vi "Measure.vi"(8 "error in (no error)":errorcluster, 9 "Progress Ref":refnum<vi>, 10 "XY Graph Reference":refnum<vi>, 11 "AM-AM in":refnum<class "AM-AM.lvclass">) -> (0 "error out":errorcluster, 2 "Results":T1[](array[typedef]), 3 "AM-AM out":refnum<class "AM-AM.lvclass">)   [LabVIEW 2020, in "AM-AM.lvclass"]
uses:
  AM-AM.lvclass
  C:/Sandbox/Git_Sandbox/WiSpry Test Framework source code (LV20)/WiSpry Test Framework/Measurements/Measurement.lvclass
  XML Handler/Controls/Result Cluster.ctl
  Path Control/Paths.ctl
  Instruments/Spectrum Analyzer/Controls/Marker Search.ctl
  AM-AM.lvclass/AM-AM.ctl
  Measurement.lvclass/Measurement.ctl
  Instruments/Spectrum Analyzer/Spectrum Analyzer.lvclass/Spectrum Analyzer.ctl
  Instruments/Spectrum Analyzer/Spectrum Analyzer.lvclass
  Instruments/Power Meter/Power Meter.lvclass
  Measurement.lvclass
  Path Control/PathControl.lvclass
  XML Handler/XML Handler.lvclass
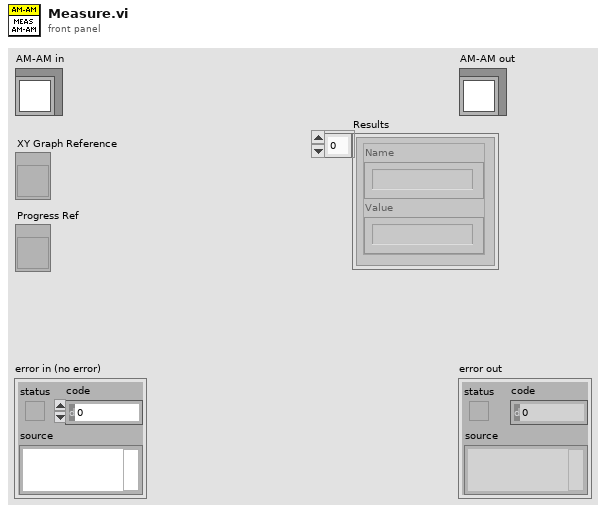
[diagram p1: front panel]
types:
  T1 = typedef "XML Handler.lvclass/Result Cluster.ctl" = cluster{"Name":string, "Value":string}
  T2 = typedef "PathControl.lvclass/Paths.ctl" = enum16{"SigGen 1 -> DUT", "SigGen 2 -> DUT", "SigGen 1 -> PM 1", "SigGen 1 -> PM 2", "DUT -> SA", "DUT -> PM 2", "VSG -> DUT", "SigGen 2 -> PM 1", "SigGen 2 -> PM 2"}
  T3 = typedef "Spectrum Analyzer.lvclass/Marker Search.ctl" = enum16{"Maximum Peak", "Maximum Next", "Maximum Right", "Maximum Left", "Minimum Peak", "Minimum Next", "Minimum Right", "Minimum Left"}
  T4 = typedef "AM-AM.lvclass/Config info.ctl" = cluster{"RBW":dbl, "VBW ":dbl, "Number of Averages":dbl, "Average On":bool, "Power":cluster{"Cluster ":cluster{"From":dbl, "To":dbl, "Step":dbl}, "Array":dbl[], "Use Array":bool}, "Frequency":cluster{"Cluster ":cluster{"From":dbl, "To":dbl, "Step":dbl}, "Array":dbl[], "Use Array":bool}, "Loop order":T5, "Power Window":dbl}
  T5 = typedef "AM-AM.lvclass/Loop order.ctl" = enum16{"Device -> Power -> Frequency", "Device -> Frequency -> Power"}
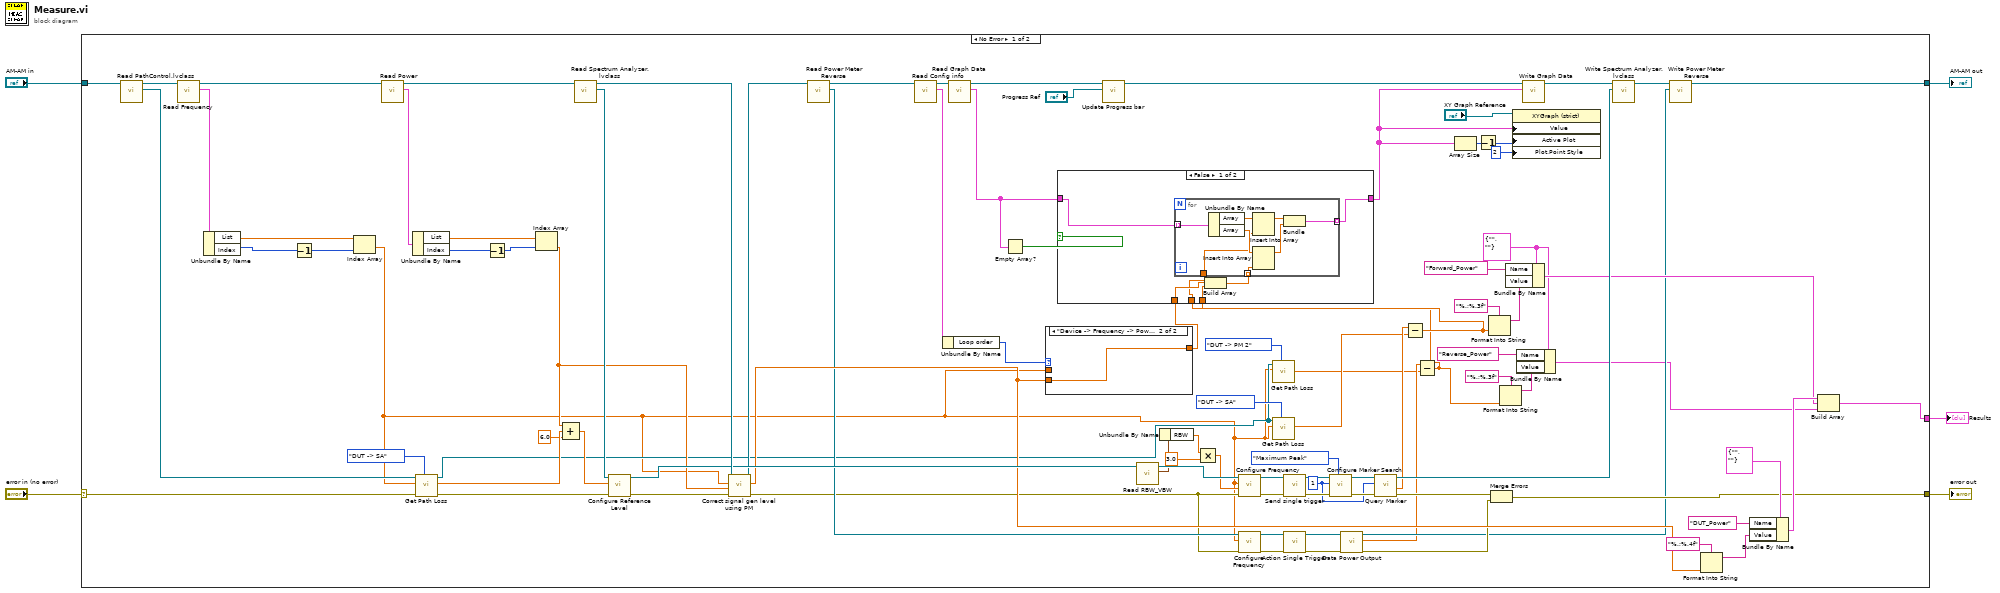
[diagram p0: block diagram]
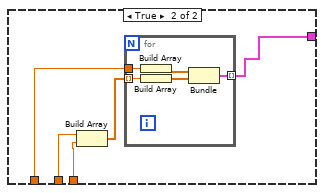
[diagram p2: hidden frame]
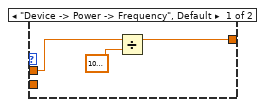
[diagram p3: hidden frame]
diagram:
  n1 = case shown="No Error" "error in (no error)" {
    selector: "error in (no error)" -> [w94 w128]
    tunnel: [w21 w128] -> w4
    tunnel: [w17 w127] -> w2
    tunnel: "AM-AM in" -> [w95 w127]
    tunnel: [w32 _] -> w1
    frame No Error {
      w8 = T1 {"Name"="", "Value"=""} ("Result Cluster")
      w47 = u32 1 ("Marker Number (1)")
      n2 = call "Read PathControl.lvclass.vi"("Measurements in"=w95) -> ("PathControl.lvclass"=w68:refnum<class "PathControl.lvclass">, "Measurements out"=w92:refnum<class "AM-AM.lvclass">)  [unwired: 9 in]
      n3 = call "Read Frequency.vi"("AM-AM in"=w92) -> ("Frequency"=w97:cluster{"List":dbl[], "Index":i32, "Last":bool}, "AM-AM out"=w98:refnum<class "AM-AM.lvclass">)  [unwired: 9 in]
      n4 = Unbundle By Name(w97) -> ("List"=w76:dbl[], "Index"=w74:i32)
      n5 = Decrement(x=w74) -> (x-1=w73:i32)
      n6 = Index Array(array=w76, index=w73) -> (element=w15:dbl)
      n7 = call "Read Power.vi"("AM-AM in"=w98) -> ("Power"=w96:cluster{"List":dbl[], "Index":i32, "Last":bool}, "AM-AM out"=w31:refnum<class "AM-AM.lvclass">)  [unwired: 9 in]
      n8 = Unbundle By Name(w96) -> ("List"=w75:dbl[], "Index"=w72:i32)
      n9 = call "Get Path Loss.vi"("Path"=Paths."DUT -> SA", "error in (no error)"=w94, "Frequency [Hz]"=w15, "PathControl in"=w68) -> ("error out"=w88:errorcluster, "Insertion Loss (dB)"=w91:dbl, "PathControl out"=w16:refnum<class "PathControl.lvclass">)  [unwired: 4 in, 1 out]
      n10 = Decrement(x=w72) -> (x-1=w71:i32)
      n11 = Index Array(array=w75, index=w71) -> (element=w66:dbl)
      n12 = Compound Arithmetic op=ADD(w66, w91, 6.0 ("value")) -> (w89:dbl)
      n13 = call "Read Spectrum Analyzer.lvclass.vi"("AM-AM in"=w31) -> ("Spectrum Analyzer.lvclass"=w90:refnum<class "Spectrum Analyzer.lvclass">, "AM-AM out"=w87:refnum<class "AM-AM.lvclass">)  [unwired: 9 in]
      n14 = call-dynamic "Configure Reference Level.vi"("error in (no error)"=w88, "Reference Level [dBm]"=w89, "Spectrum Analyzer in"=w90) -> ("error out"=w67:errorcluster, "Spectrum Analyzer out"=w86:refnum<class "Spectrum Analyzer.lvclass">)  [unwired: 7 in]
      n15 = call "Correct signal gen level using PM.vi"("error in (no error)"=w67, "Power"=w66, "Frequency"=w15, "AM-AM in"=w87) -> ("error out"=w26:errorcluster, "Power at DUT"=w61:dbl, "AM-AM out"=w29:refnum<class "AM-AM.lvclass">)  [unwired: 5 in]
      n16 = call "Read Power Meter Reverse.vi"("AM-AM in"=w29) -> ("Power Meter.lvclass"=w27:refnum<class "Power Meter.lvclass">, "AM-AM out"=w28:refnum<class "AM-AM.lvclass">)  [unwired: 9 in]
      n17 = call "Read Config info.vi"("AM-AM in"=w28) -> ("Config info"=w82:T4, "AM-AM out"=w83:refnum<class "AM-AM.lvclass">)  [unwired: 9 in]
      n18 = Unbundle By Name(w82) -> ("Loop order"=w81:T5)
      n19 = call "Read Graph Data.vi"("AM-AM in"=w83) -> ("Graph Data"=w70:cluster{"Array":dbl[], "Array":dbl[]}[], "AM-AM out"=w78:refnum<class "AM-AM.lvclass">)  [unwired: 9 in]
      n20 = Empty Array?(array=w70) -> (empty?=w69:bool)
      n21 = case shown="\"Device -> Frequency -> Power\"" w81 {
        tunnel: w15 -> [w125 _]
        tunnel: w61 -> [_ w126]
        tunnel: [w124 w126] -> w41
        frame "Device -> Power -> Frequency", Default {
          n22 = Divide(x=w125, y=1000000.0) -> (x/y=w124:dbl)
        }
        frame "Device -> Frequency -> Power" {
        }
      }
      n23 = call "Update Progress bar.vi"("Progress Ref"="Progress Ref", "Measurements In"=w78) -> ("Measurements Out"=w77:refnum<class "AM-AM.lvclass">)  [unwired: 9 in]
      n24 = call "Read RBW_VBW.vi"("Spectrum Analyzer in"=w86) -> ("RBW/VBW"=w59:cluster{"RBW":dbl, "VBW":dbl}, "Spectrum Analyzer out"=w60:refnum<class "Spectrum Analyzer.lvclass">)  [unwired: 9 in]
      n25 = Unbundle By Name(w59) -> ("RBW"=w58:dbl)
      n26 = Multiply(x=w58, y=3.0) -> (x*y=w56:dbl)
      n27 = call-dynamic "Configure Frequency.vi"("error in (no error)"=w26, "Span/Stop Frequency [Hz]"=w56, "Center/Start Frequency [Hz]"=w15, "Spectrum Analyzer in"=w60) -> ("error out"=w55:errorcluster, "Spectrum Analyzer out"=w54:refnum<class "Spectrum Analyzer.lvclass">)  [unwired: 6 in]
      n28 = call-dynamic "Configure Frequency.vi"("error in (no error)"=w26, "Frequency"=w15, "Power Meter in"=w27) -> ("error out"=w25:errorcluster, "Power Meter out"=w24:refnum<class "Power Meter.lvclass">)  [unwired: 7 in]
      n29 = call "Get Path Loss.vi"("Path"=Paths."DUT -> PM 2", "Frequency [Hz]"=w15, "PathControl in"=w16) -> ("Insertion Loss (dB)"=w12:dbl)  [unwired: 5 in, 3 out]
      n30 = call "Get Path Loss.vi"("Path"=Paths."DUT -> SA", "Frequency [Hz]"=w15, "PathControl in"=w16) -> ("Insertion Loss (dB)"=w43:dbl)  [unwired: 5 in, 3 out]
      n31 = call-dynamic "Send single trigger.vi"("error in (no error)"=w55, "Spectrum Analyzer in"=w54) -> ("error out"=w52:errorcluster, "Spectrum Analyzer out"=w51:refnum<class "Spectrum Analyzer.lvclass">)  [unwired: 8 in]
      n32 = call-dynamic "Action Single Trigger.vi"("error in (no error)"=w25, "Power Meter in"=w24) -> ("error out"=w22:errorcluster, "Power Meter out"=w23:refnum<class "Power Meter.lvclass">)  [unwired: 8 in]
      n33 = call-dynamic "Configure Marker Search.vi"("Marker Search (Max Peak)"=Marker_Search."Maximum Peak", "error in (no error)"=w52, "Marker Number (1)"=w47, "Spectrum Analyzer in"=w51) -> ("error out"=w49:errorcluster, "Spectrum Analyzer out"=w48:refnum<class "Spectrum Analyzer.lvclass">)  [unwired: 6 in]
      n34 = call-dynamic "Data Power Output.vi"("error in (no error)"=w22, "Power Meter in"=w23) -> ("error out"=w20:errorcluster, "Power Out"=w13:dbl, "Power Meter out"=w18:refnum<class "Power Meter.lvclass">)  [unwired: 7 in]
      n35 = call-dynamic "Query Marker.vi"("error in (no error)"=w49, "Marker Number (1)"=w47, "Spectrum Analyzer in"=w48) -> ("error out"=w85:errorcluster, "Marker Level"=w44:dbl, "Spectrum Analyzer out"=w84:refnum<class "Spectrum Analyzer.lvclass">)  [unwired: 5 in, 1 out]
      n36 = Subtract(x=w44, y=w43) -> (x-y=w42:dbl)
      n37 = Subtract(x=w13, y=w12) -> (x-y=w6:dbl)
      n38 = case shown="False" w69 {
        tunnel: w42 -> [w102 w116]
        tunnel: w41 -> [w104 w117]
        tunnel: w70 -> [w103 _]
        tunnel: [w99 w113] -> w79
        tunnel: w6 -> [w101 w115]
        frame False {
          n39 = Build Array(w102, w101) -> (w100:dbl[])
          n40 = for {
            tunnel: w104 -> [w110]
            tunnel: w103 -> [w107] mode=indexing
            tunnel: w100 -> [w106] mode=indexing
            tunnel: [w105] -> w99 mode=indexing
            n41 = Unbundle By Name(w107) -> ("Array"=w112:dbl[], "Array"=w111:dbl[])
            n42 = Insert Into Array(array=w112, new element=w110) -> (w109:dbl[])  [unwired: 1 in]
            n43 = Insert Into Array(array=w111, new element=w106) -> (w108:dbl[])  [unwired: 1 in]
            n44 = Bundle("Array"=w109, "Array"=w108) -> (w105:cluster{"Array":dbl[], "Array":dbl[]})  [unwired: 1 in]
          }
        }
        frame True {
          n45 = Build Array(w116, w115) -> (w114:dbl[])
          n46 = for {
            tunnel: w117 -> [w122]
            tunnel: w114 -> [w119] mode=indexing
            tunnel: [w118] -> w113 mode=indexing
            n47 = Build Array(w122) -> (w121:dbl[])
            n48 = Build Array(w119) -> (w120:dbl[])
            n49 = Bundle(w121, w120) -> (w118:cluster{dbl[], dbl[]})  [unwired: 1 in]
          }
        }
      }
      n50 = Array Size(array=w79) -> (size(s)=w38:i32)
      n51 = Decrement(x=w38) -> (x-1=w37:i32)
      n52 = Format Into String(format string="%.;%.3f", w42) -> (resulting string=w46:string)  [unwired: 2 in, 1 out]
      n53 = Merge Errors(w85, w20) -> (w21:errorcluster)
      n54 = Format Into String(format string="%.;%.3f", w6) -> (resulting string=w10:string)  [unwired: 2 in, 1 out]
      n55 = Bundle By Name(cluster=w8, "Name"="Forward_Power" ("format string"), "Value"=w46) -> (w33:T1)
      n56 = property class="XYGraph (strict)"(reference="XY Graph Reference", "Value"=w79, "Active Plot"=w37, "Plot.Point Style"=u8 2) -> ()  [unwired: 1 in, 2 out]
      n57 = Bundle By Name(cluster=w8, "Name"="Reverse_Power" ("format string"), "Value"=w10) -> (w7:T1)
      n58 = call "Write Graph Data.vi"("Graph Data"=w79, "AM-AM in"=w77) -> ("AM-AM out"=w80:refnum<class "AM-AM.lvclass">)  [unwired: 9 in]
      n59 = call "Write Spectrum Analyzer.lvclass.vi"("Spectrum Analyzer.lvclass"=w84, "AM-AM in"=w80) -> ("AM-AM out"=w19:refnum<class "AM-AM.lvclass">)  [unwired: 9 in]
      n60 = call "Write Power Meter Reverse.vi"("Power Meter.lvclass"=w18, "AM-AM in"=w19) -> ("AM-AM out"=w17:refnum<class "AM-AM.lvclass">)  [unwired: 9 in]
      n61 = Format Into String(format string="%.;%.4f", w61) -> (resulting string=w62:string)  [unwired: 2 in, 1 out]
      n62 = Bundle By Name(cluster=T1 {"Name"="", "Value"=""} ("new element/subarray"), "Name"="DUT_Power", "Value"=w62) -> (w34:T1)
      n63 = Build Array(w34, w33, w7) -> (w32:T1[])
    }
    frame Error {
    }
  }
  "error out" <- w4
  "AM-AM out" <- w2
  "Results" <- w1
